vi "Add VIs to Class.vi"(8 "error in (no error)":errorcluster, 9 "Folder Name":string="APIs", 10 "DVR VI Paths[]":path[](array[path]), 11 "Class Path":path=path "D:/GitHub/LabVIEW/SLL/Tools/Class DVR API Generator/Example/My Sample Class.lvclass") -> (0 "error out":errorcluster)   [LabVIEW 2016, in "SLL Class DVR API Generator.lvlib"]
uses:
  SLL Class DVR API Generator.lvlib
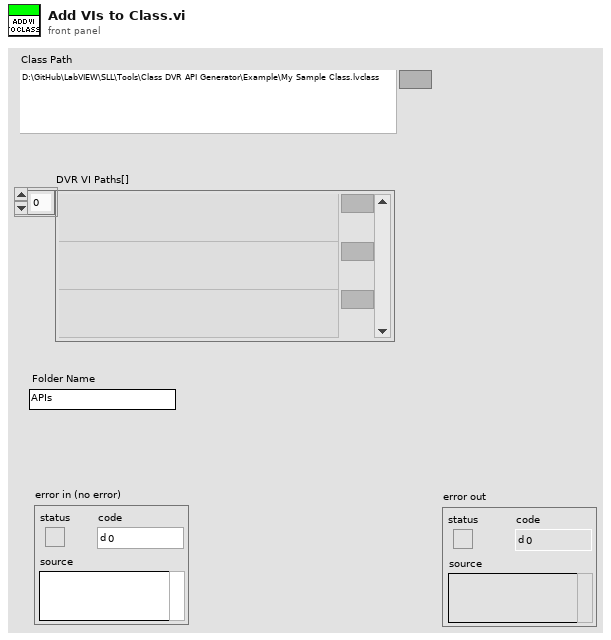
[diagram p1: front panel]
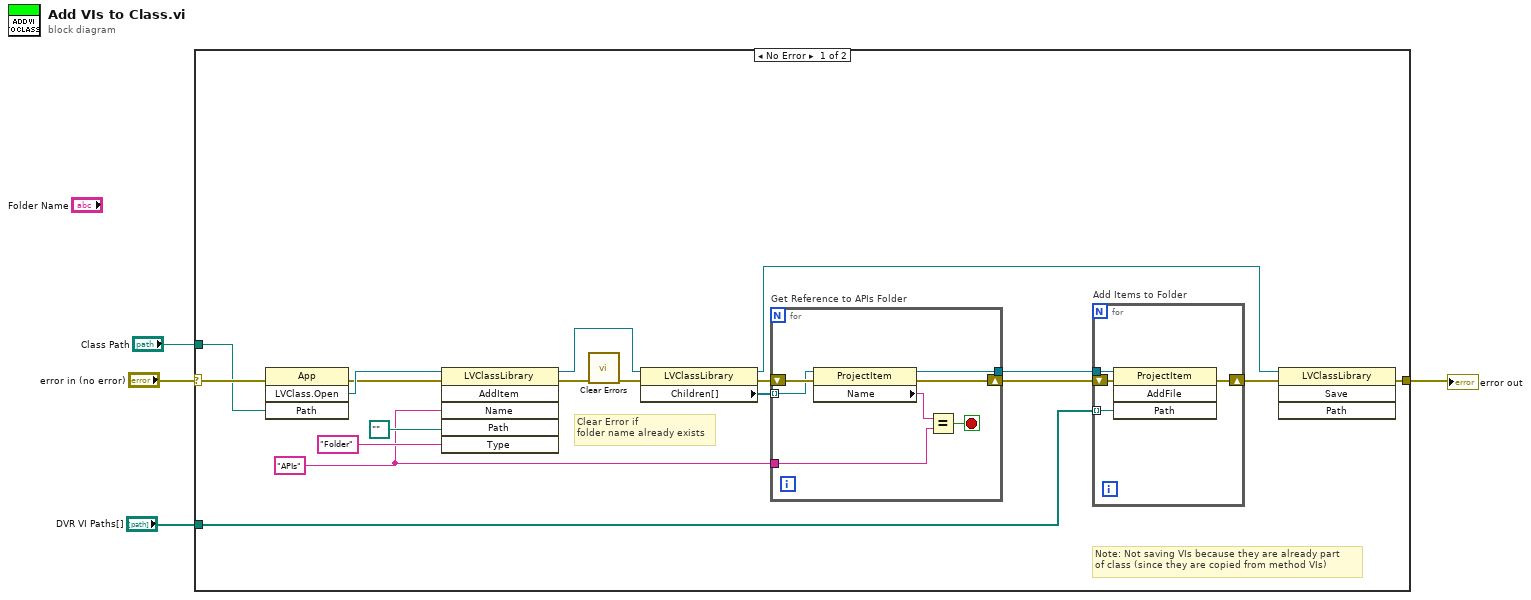
[diagram p0: block diagram]
diagram:
  n1 = case shown="No Error" "error in (no error)" {
    selector: "error in (no error)" -> [w22 w34]
    tunnel: [w6 w34] -> w3
    tunnel: "Class Path" -> [w21 _]
    tunnel: "DVR VI Paths[]" -> [w7 _]
    frame No Error {
      w10 = "APIs" ("Name")
      # "Note: Not saving VIs because they are already part \nof class (since they are copied from method VIs)"
      # "Clear Error if \nfolder name already exists"
      n2 = invoke class="App" method="LVClass.Open"(error in=w22, "Path"=w21) -> (error out=w16:errorcluster, "LVClass.Open"=w18:refnum<vi>)  [unwired: 2 in, 2 out]
      n3 = invoke class="LVClassLibrary" method="AddItem"(reference=w18, error in=w16, "Name"=w10, "Path"=path "", "Type"="Folder") -> (reference out=w13:refnum<vi>, error out=w20:errorcluster)  [unwired: 1 in, 4 out]
      n4 = call <vilib>:"Clear Errors.vi"("error in (no error)"=w20) -> ("error out"=w15:errorcluster)  [unwired: 5 in, 1 out]
      n5 = property class="LVClassLibrary"(reference=w13, error in=w15) -> (reference out=w5:refnum<vi>, error out=w14:errorcluster, "Children[]"=w11:refnum<vi>[])
      n6 = for "Get Reference to APIs Folder" {
        shift-right: [w32] -> w12
        shift-left: w14 -> [w33]
        tunnel: w11 -> [w31] mode=indexing
        tunnel: w10 -> [w29]
        tunnel: [w27] -> w8
        stop <- w28 stop-if-true
        n7 = property class="ProjectItem"(reference=w31, error in=w33) -> (reference out=w27:refnum<vi>, error out=w32:errorcluster, "Name"=w30:string)
        n8 = Equal?(x=w30, y=w29) -> (x = y?=w28:bool)
      }
      n9 = for "Add Items to Folder" {
        tunnel: w8 -> [w24]
        shift-right: [w25] -> w9
        shift-left: w12 -> [w26]
        tunnel: w7 -> [w23] mode=indexing
        n10 = invoke class="ProjectItem" method="AddFile"(reference=w24, error in=w26, "Path"=w23) -> (error out=w25:errorcluster)  [unwired: 1 in, 3 out]
      }
      n11 = invoke class="LVClassLibrary" method="Save"(reference=w5, error in=w9) -> (error out=w6:errorcluster)  [unwired: 2 in, 3 out]
    }
    frame Error {
    }
  }
  "error out" <- w3
